vi "test_drop.vi"() -> ()   [LabVIEW 2015]
panel:
  out "regex":string
  in  "stop":bool
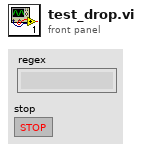
[diagram p1: front panel]
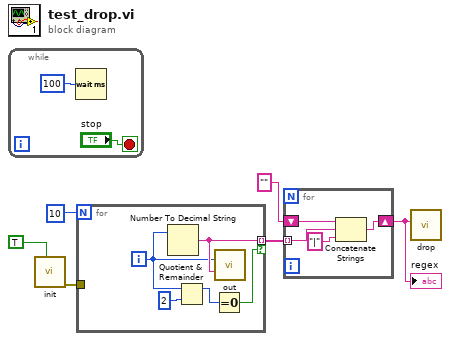
[diagram p0: block diagram]
diagram:
  n1 = while {
    stop <- "stop" stop-if-true
    n2 = Wait (ms)(milliseconds to wait=u32 100) -> ()  [unwired: 1 out]
  }
  n3 = call "init.vi"("Cleaneup"=TRUE) -> ("error out"=w2:errorcluster)  [unwired: 10 in]
  n4 = for {
    N: 10 -> [_]
    tunnel: [w10] -> w5 mode=indexing if=w11
    tunnel: w2 -> [_]
    i -> [w9]
    n5 = Number To Decimal String(number=w9) -> (decimal integer string=w10:string)  [unwired: 1 in]
    n6 = Quotient & Remainder(x=w9, y=2) -> (x-y*floor(x/y)=w12:i32)  [unwired: 1 out]
    n7 = Equal To 0?(x=w12) -> (x = 0?=w11:bool)
    n8 = call "out.vi"("IN VARIANT"=w9, "Name in"=w10) -> ()  [unwired: 12 in, 2 out]
  }
  n9 = for {
    tunnel: w5 -> [w14] mode=indexing
    shift-right: [w17] -> w4
    shift-left: "" -> [w16]
    n10 = Concatenate Strings(w16, w14, "|" ("string")) -> (w17:string)
  }
  "regex" <- w4
  n11 = call "drop.vi"("Regex"=w4) -> ()  [unwired: 10 in, 1 out]
